vi "niScope Fetch Measurement (poly).vi"   [LabVIEW 2013]
doc: "Obtains a waveform from the digitizer and returns the specified measurement."
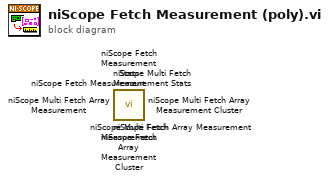
[diagram p0: block diagram]
diagram:
  n1 = call <instrlib>:"niScope Multi Fetch Measurement.vi"() -> ()  [unwired: 13 in, 3 out]
  n2 = call <instrlib>:"niScope Multi Fetch Measurement Stats.vi"() -> ()  [unwired: 13 in, 3 out]
  n3 = call <instrlib>:"niScope Multi Fetch Array Measurement.vi"() -> ()  [unwired: 12 in, 4 out]
  n4 = call <instrlib>:"niScope Multi Fetch Array Measurement Cluster.vi"() -> ()  [unwired: 12 in, 4 out]
  n5 = call <instrlib>:"niScope Fetch Measurement.vi"() -> ()  [unwired: 13 in, 3 out]
  n6 = call <instrlib>:"niScope Fetch Measurement Stats.vi"() -> ()  [unwired: 13 in, 3 out]
  n7 = call <instrlib>:"niScope Fetch Array Measurement.vi"() -> ()  [unwired: 12 in, 4 out]
  n8 = call <instrlib>:"niScope Fetch Array Measurement Cluster.vi"() -> ()  [unwired: 12 in, 4 out]
